vi "Settings_Widefield.vi"() -> ()   [LabVIEW 2012]
uses:
  <vilib>/Utility/file.llb/Read From Spreadsheet File (DBL).vi
  Widefield_globals.vi
panel:
  in  "Camera Type":u16(ring) items=["AVT Manta", "Hamamatsu Orca", "Hamamatsu Orca2"]
  in  "FOV size (um)":i32[](array[numeric])=[2000, 1500]
  in  "Binning":u16(ring) items=["1X1", "2X2", "4X4", "8X8"]
  out "Frames":i32
  in  "Frame Offset":i32
  in  "Both bulbs|One bulb?":bool
  in  "LED Settle time (ms)":i32=500
  in  "Odor Build Up (ms)":i32
  in  "Continuous|Timer?":bool
  in  "Frame rate (Hz)":dbl=8.9 min=1.0 max=8.9
  out "FrameTime (ms)":i32=112
  in  "Control LED?":bool
  in  "ITI (ms)":i32=30000
  in  "Randomize?":bool
  in  "Save single frames?":bool=TRUE
  out "Exposure (ms)":dbl=112.0
  in  "Y":i32=4
  in  "X":i32=4
  in  "File path (for saving data)":path
  in  "# Repeats":u16=5 min=1 max=1000
  in  "Done!":bool
  # "Acquisition settings"
  # "Stimulus settings"
  # "For Timer mode only"
  # "Binning"
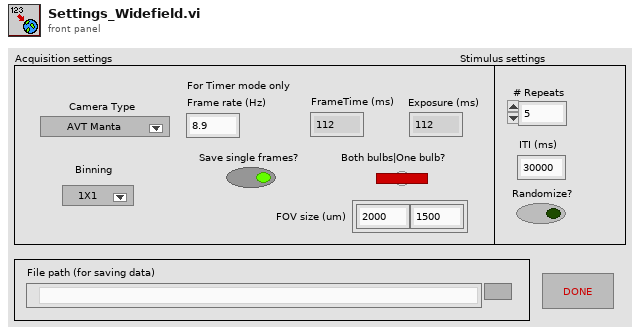
[diagram p1: front panel]
types:
  T1 = typedef "LVStringsAndValuesArrayTypeDef_U16.ctl" = cluster{"String":string, "Value":u16}[]
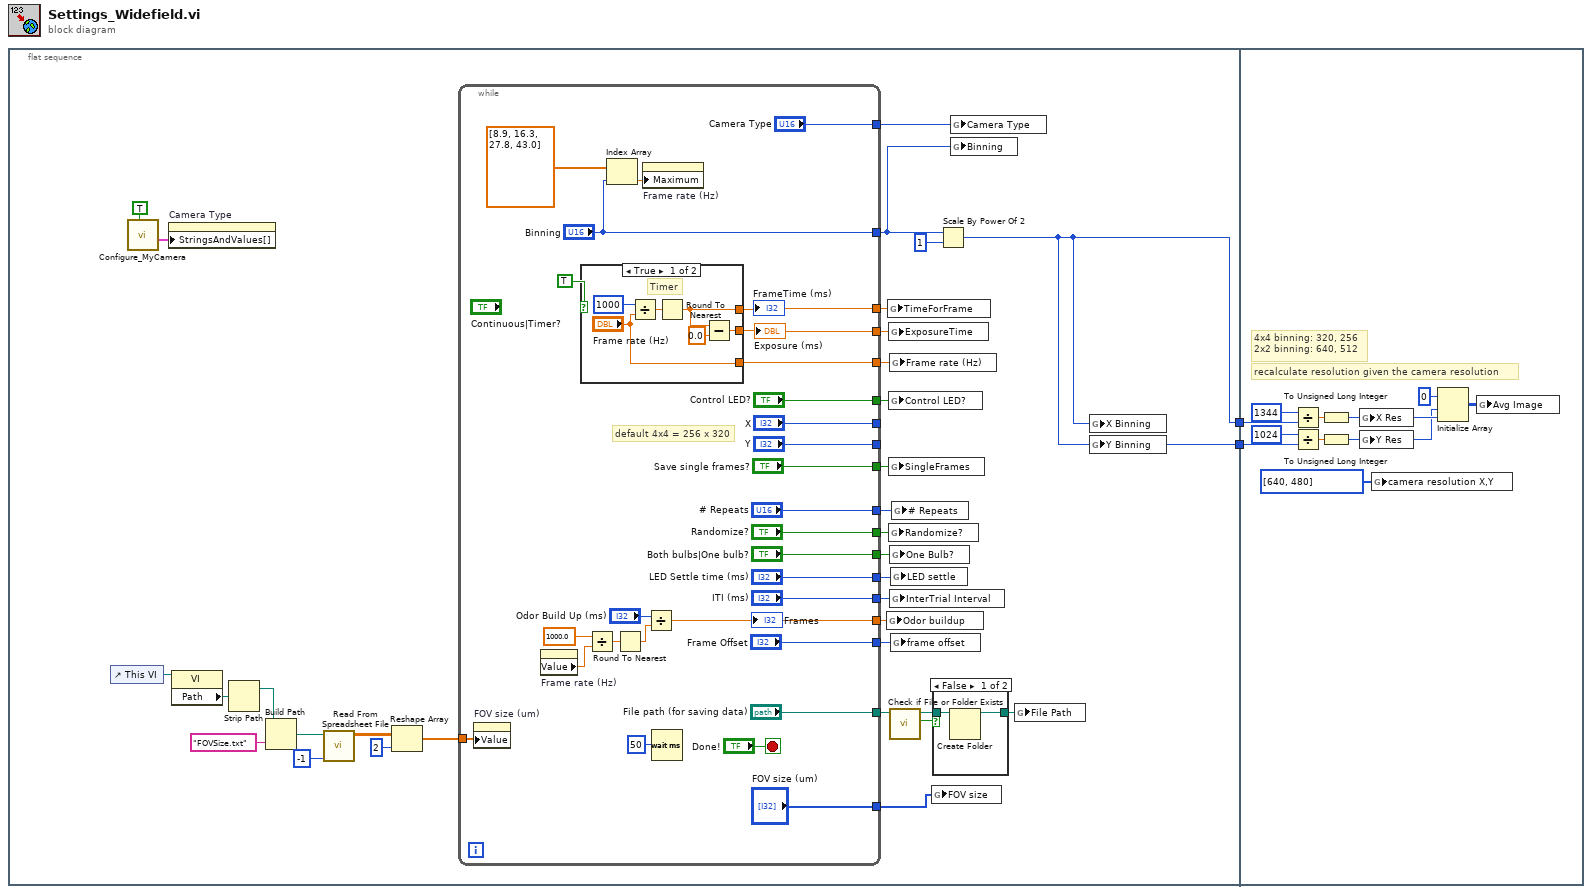
[diagram p0: block diagram]
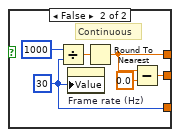
[diagram p3: hidden frame]
diagram:
  n1 = flat-sequence {
    tunnel: [w21] -> w2
    tunnel: [w21] -> w1
    tunnel: w1 -> [w82]
    tunnel: w2 -> [w83]
    frame #0 {
      n2 = control-ref of="This VI"() -> (w15:refnum<vi>)
      n3 = call "Configure_MyCamera.vi"("Get Camera Types"=TRUE) -> ("Camera Types"=w3:T1)  [unwired: 5 in, 2 out]
      n4 = property on="Camera Type" class="Ring (strict)"("StringsAndValues[]"=w3) -> ()  [unwired: 2 in, 2 out]
      n5 = property class="VI"(reference=w15) -> ("Path"=w14:path)  [unwired: 1 in, 2 out]
      n6 = Strip Path(path=w14) -> (stripped path=w13:path)  [unwired: 1 out]
      n7 = Build Path(base path=w13, name or relative path="FOVSize.txt") -> (appended path=w11:path)
      n8 = call-poly <vilib>:"Read From Spreadsheet File.vi"("number of rows (all:-1)"=-1, "file path (dialog if empty)"=w11) -> ("all rows"=w9:dbl[][])  [unwired: 5 in, 4 out]
      n9 = Reshape Array(w9, 2 ("dimension size")) -> (w7:dbl[])
      n10 = while {
        tunnel: [w64] -> w34
        tunnel: [w63] -> w33
        tunnel: ["X"] -> _
        tunnel: ["Y"] -> _
        tunnel: ["Save single frames?"] -> w32
        tunnel: ["Control LED?"] -> w31
        tunnel: ["# Repeats"] -> w30
        tunnel: ["Randomize?"] -> w29
        tunnel: ["ITI (ms)"] -> w28
        tunnel: ["File path (for saving data)"] -> w19
        tunnel: ["Both bulbs|One bulb?"] -> w27
        tunnel: ["LED Settle time (ms)"] -> w26
        tunnel: [w53] -> w25
        tunnel: ["Frame Offset"] -> w24
        tunnel: [w45] -> w23
        tunnel: ["Binning"] -> w20
        tunnel: w7 -> [w41]
        tunnel: ["FOV size (um)"] -> w6
        tunnel: ["Camera Type"] -> w5
        stop <- "Done!" stop-if-true
        # "default 4x4 = 256 x 320"
        n11 = property on="FOV size (um)" class="Arr (strict)"("Value"=w41) -> ()  [unwired: 2 in, 2 out]
        n12 = property on="Frame rate (Hz)" class="DigNum (strict)"() -> ("Value"=w50:dbl)  [unwired: 2 in, 2 out]
        n13 = case shown="True" TRUE {
          tunnel: [w70 w76] -> w64
          tunnel: [w69 w75] -> w63
          tunnel: ["Frame rate (Hz)" w73] -> w53
          frame True {
            # "Timer"
            n14 = Divide(x=1000, y="Frame rate (Hz)") -> (x/y=w71:dbl)
            n15 = Round To Nearest(number=w71) -> (nearest integer value=w70:dbl)
            n16 = Subtract(x=w70, y=0.0) -> (x-y=w69:dbl)
          }
          frame False {
            w73 = 30 ("Frame rate (Hz) 2")
            # "Continuous"
            n17 = Divide(x=1000, y=w73) -> (x/y=w77:dbl)
            n18 = property on="Frame rate (Hz)" class="DigNum (strict)"("Value"=w73) -> ()  [unwired: 2 in, 2 out]
            n19 = Round To Nearest(number=w77) -> (nearest integer value=w76:dbl)
            n20 = Subtract(x=w76, y=0.0) -> (x-y=w75:dbl)
          }
        }
        "Exposure (ms)" <- w63
        "FrameTime (ms)" <- w64
        n21 = Divide(x=1000.0, y=w50) -> (x/y=w47:dbl)
        n22 = Index Array(array=dbl[] [8.9, 16.3, 27.8, 43.0], index="Binning") -> (element=w43:dbl)
        n23 = Round To Nearest(number=w47) -> (nearest integer value=w48:dbl)
        n24 = property on="Frame rate (Hz)" class="DigNum (strict)"("Maximum"=w43) -> ()  [unwired: 2 in, 2 out]
        n25 = Divide(x="Odor Build Up (ms)", y=w48) -> (x/y=w45:dbl)
        "Frames" <- w45
        n26 = Wait (ms)(milliseconds to wait=50) -> ()  [unwired: 1 out]
      }
      n27 = global write "Widefield_globals.vi" "Odor buildup"(w23) -> ()
      n28 = global write "Widefield_globals.vi" "TimeForFrame"(w34) -> ()
      n29 = global write "Widefield_globals.vi" "ExposureTime"(w33) -> ()
      n30 = global write "Widefield_globals.vi" "Control LED?"(w31) -> ()
      n31 = global write "Widefield_globals.vi" "SingleFrames"(w32) -> ()
      n32 = global write "Widefield_globals.vi" "Randomize?"(w29) -> ()
      n33 = global write "Widefield_globals.vi" "Frame rate (Hz)"(w25) -> ()
      n34 = global write "Widefield_globals.vi" "One Bulb?"(w27) -> ()
      n35 = global write "Widefield_globals.vi" "InterTrial Interval"(w28) -> ()
      n36 = call <vilib>:"Check if File or Folder Exists.vi"("path"=w19) -> ("file or folder exists?"=w18:bool, "dup path"=w17:path)  [unwired: 8 in, 1 out]
      n37 = global write "Widefield_globals.vi" "LED settle"(w26) -> ()
      n38 = global write "Widefield_globals.vi" "frame offset"(w24) -> ()
      n39 = global write "Widefield_globals.vi" "# Repeats"(w30) -> ()
      n40 = global write "Widefield_globals.vi" "FOV size"(w6) -> ()
      n41 = case shown="False" w18 {
        tunnel: [w35 w37] -> w16
        tunnel: w17 -> [w36 w37]
        frame False {
          n42 = Create Folder(path (use dialog)=w36) -> (created path=w35:path)  [unwired: 2 in, 2 out]
        }
        frame True {
        }
      }
      n43 = Scale By Power Of 2(n=w20, x=u16 1) -> (x*2^n=w21:u16)
      n44 = global write "Widefield_globals.vi" "Camera Type"(w5) -> ()
      n45 = global write "Widefield_globals.vi" "Binning"(w20) -> ()
      n46 = global write "Widefield_globals.vi" "File Path"(w16) -> ()
      n47 = global write "Widefield_globals.vi" "X Binning"(w21) -> ()
      n48 = global write "Widefield_globals.vi" "Y Binning"(w21) -> ()
    }
    frame #1 {
      # "4x4 binning: 320, 256 \n2x2 binning: 640, 512"
      # "recalculate resolution given the camera resolution"
      n49 = Divide(x=1344, y=w83) -> (x/y=w89:dbl)
      n50 = Divide(x=1024, y=w82) -> (x/y=w88:dbl)
      n51 = To Unsigned Long Integer(number=w89) -> (unsigned 32bit integer=w81:u32)
      n52 = To Unsigned Long Integer(number=w88) -> (unsigned 32bit integer=w80:u32)
      n53 = global write "Widefield_globals.vi" "X Res"(w81) -> ()
      n54 = global write "Widefield_globals.vi" "Y Res"(w80) -> ()
      n55 = global write "Widefield_globals.vi" "camera resolution X,Y"(i32[] [640, 480] ("camera resolution X,Y")) -> ()
      n56 = Initialize Array(u16 0 ("element"), w80, w81) -> (w84:u16[][])
      n57 = global write "Widefield_globals.vi" "Avg Image"(w84) -> ()
    }
  }
